vi "Robot Global Data.vi"() -> ()   [LabVIEW 2017]
doc: "This global VI can contain as many global variables as you need. To create a global variable, place a control on the panel, give it a good name. To read or write to it from a VI, drag the icon to the diagram of that VI. You can also drag from the project. Click on the node to change which global you access. You shouldn't have multiple locations writing to a global or it will cause a race-condition."
uses:
  <vilib>/Rock Robotics/WPI/Camera/WPI_CameraImageSize.ctl
  <vilib>/Rock Robotics/WPI/DriverStation/WPI_DriverStationRobotMode2.ctl
panel:
  out "DriveXAxisCorrection":dbl
  out "UseLDriveEncoder":bool
  out "LDriveEncoder":i32
  out "ArmSwitch":bool
  out "ArmEncoder":i32
  out "BellySensor":bool
  out "ArmSensor":bool
  out "RDriveEncoder":i32
  out "GyroReset":bool
  out "GyroHeading":dbl
  out "ImmedaiteModeEnable":bool
  out "TeamColorRed":bool
  out "RivalSwitchLeft":bool
  out "TeamScaleLeft":bool
  out "TeamSwitchLeft":bool
  out "FlipControls":bool
  in  "Robot Mode":T1
  in  "image size":T2=enum."320x240"
  in  "Enable Vision":bool
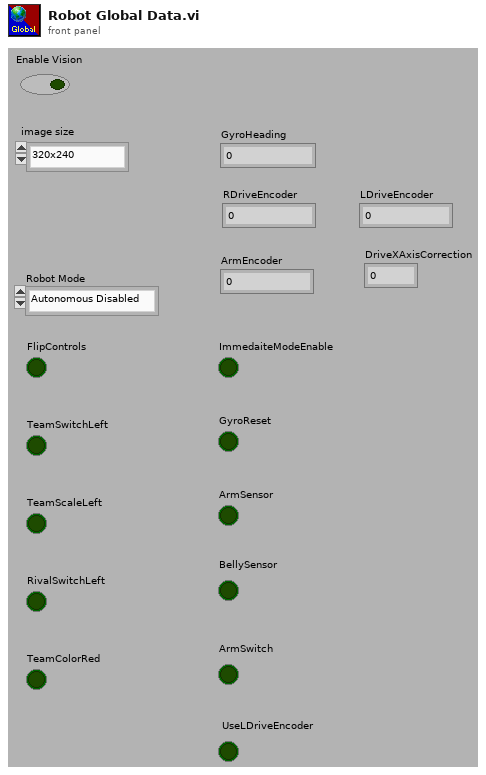
[diagram p1: front panel]
types:
  T1 = typedef "WPI_DriverStationRobotMode2.ctl" = enum16{"Autonomous Disabled", "Autonomous Enabled", "Teleop Disabled", "Teleop Enabled", "Disconnected", "Finish", "Test Disabled", "Test Enabled", "Emergency Stopped"}
  T2 = typedef "WPI_CameraImageSize.ctl" = enum16{"640x480", "320x240", "160x120", "Custom"}
diagram:
